vi "Express VI - Spectral Measurements.vi"() -> ()   [LabVIEW 2023]
doc: "This example shows how to take a spectral measurement on a simulated signal. The spectral measurement is a Peak FFT of the simulated signal.\n\nThis example uses the following Express VIs: Simulate Signal and Spectral Measurements."
uses:
  Instance           2 34Saved   Basic Spectral Measurement .vi
  <vilib>/express/express analysis/Spectral/Block/exnSpectralBlock spectral measurements peak poly.vi
  <vilib>/express/express analysis/Spectral/Block/exnSpectralBlock spectral measurements peak DDT.vi
  <vilib>/express/express analysis/Spectral/XNode/ExpressSpectralMeasurementsBlockNode.xnode
panel:
  in  "Frequency":dbl(slide)=100.0 scale=0.0..400.0
  out "Input":dynamicdata(graph)
  in  "Stop":bool
  out "Result":dynamicdata(graph)
  # "Overview: Demonstrates how to take a spectral measurement on a simulated signal.\nRequirements: LabVIEW Full Development System\nInstructions:\n1. Run the VI.\n2. Change the Frequency with the slider.\n3. Click Stop to stop the VI.\n4. Open the block diagram, right click on the Spectral Measurements Express VI and select Properties to explore the configuration options."
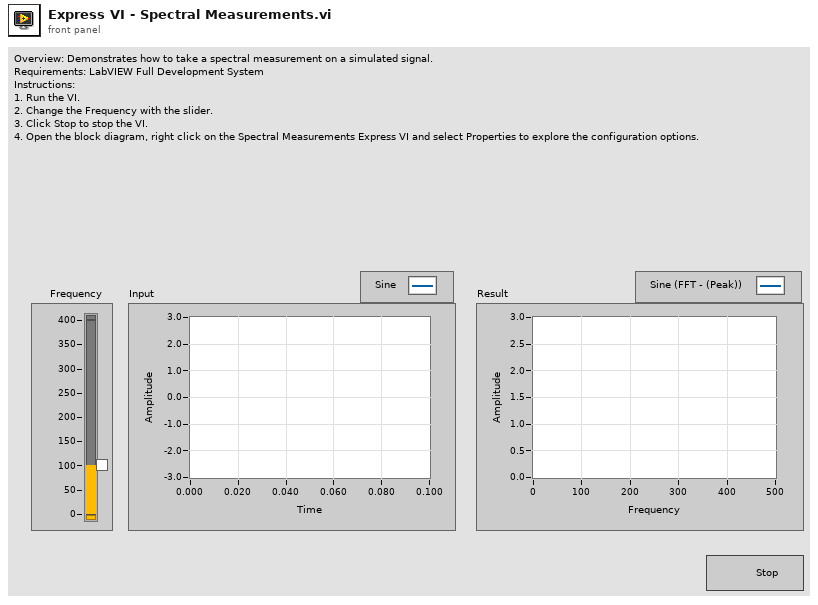
[diagram p1: front panel]
types:
  T1 = cluster{"averaging mode":u16, "weighting mode":u16, "number of averages":u32}
  T2 = cluster{"dB On (F)":bool, "unwrap phase (F)":bool, "convert to degree (F)":bool}
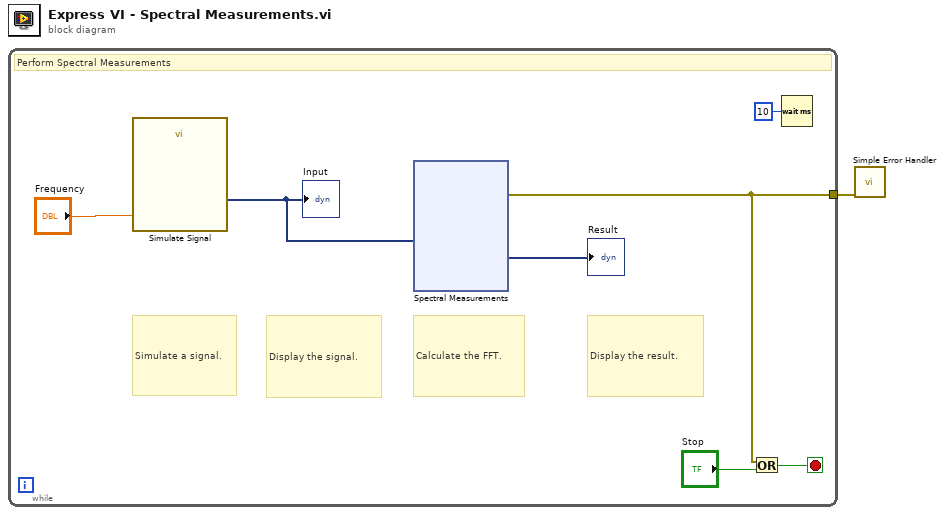
[diagram p0: block diagram]
diagram:
  n1 = while {
    tunnel: [w2] -> w1
    stop <- w3 stop-if-true
    # "Display the result."
    # "Calculate the FFT."
    # "Display the signal."
    # "Simulate a signal."
    # "Perform Spectral Measurements"
    n2 = call "Simulate Signal"("Frequency"="Frequency") -> ("Sine"=w6:dynamicdata)  [unwired: 5 in, 9 out]
    "Input" <- w6
    n3 = xnode "Spectral Measurements"("Signals"=w6) -> ("FFT - (Peak)"=→"Result":dynamicdata, "error out"=w2:errorcluster)  [unwired: 1 in, 1 out]
    n4 = Or(x=w2, y="Stop") -> (x .or. y?=w3:bool)
    n5 = Wait (ms)(milliseconds to wait=u32 10) -> ()  [unwired: 1 out]
  }
  n6 = call <vilib>:"Simple Error Handler.vi"("error in (no error)"=w1) -> ()  [unwired: 4 in, 5 out]
